vi "bluetooth com template.vi"   [LabVIEW 2021]
uses:
  <vilib>/Aledyne-TSXperts/Arduino Compatible Compiler for LabVIEW/Code Generator/Arduino APIs/Digital/PinDirection.ctl
  <vilib>/Aledyne-TSXperts/Arduino Compatible Compiler for LabVIEW/Code Generator/Arduino APIs/Serial/Serial Settings.ctl
  <vilib>/Aledyne-TSXperts/Arduino Compatible Compiler for LabVIEW/Arduino Compatible Compiler for LabVIEW.lvlib
types:
  T1 = typedef "Arduino Compatible Compiler for LabVIEW.lvlib/PinDirection.ctl" = enum16{" INPUT", "OUTPUT", " INPUT_PULLUP"}
  T2 = typedef "Arduino Compatible Compiler for LabVIEW.lvlib/Serial Settings.ctl" = u16
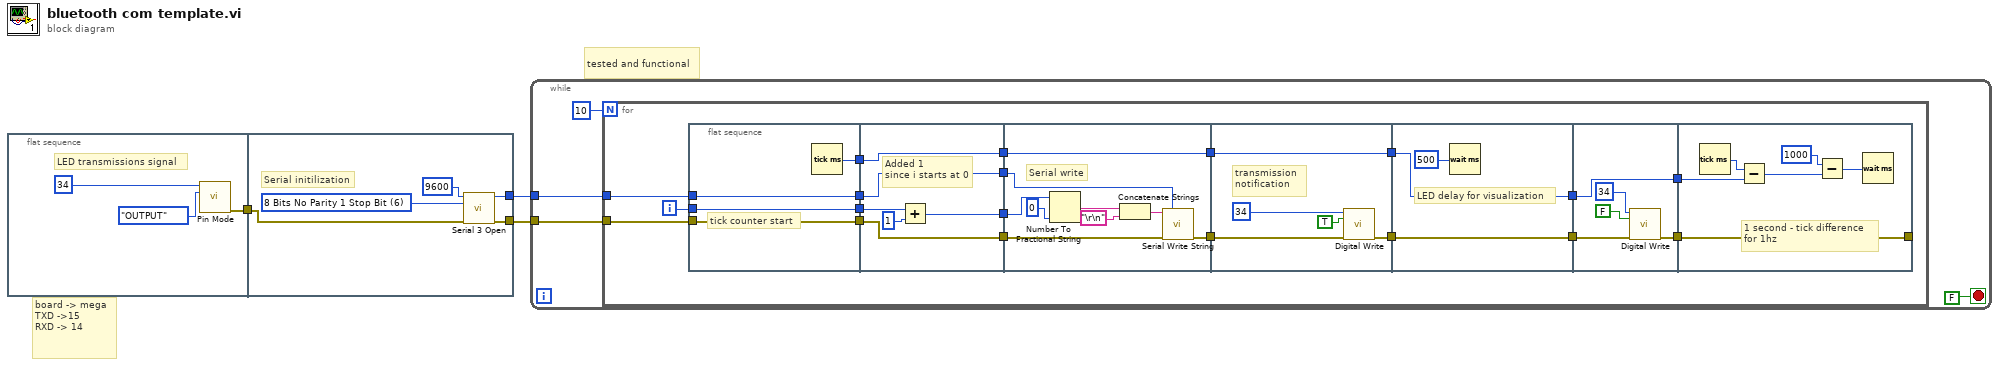
[diagram p0: block diagram]
diagram:
  # "tested and functional"
  # "board -> mega\nTXD ->15\nRXD -> 14"
  n1 = flat-sequence {
    tunnel: [w4] -> w3
    tunnel: [w11] -> w1
    tunnel: [w10] -> w2
    tunnel: w3 -> [w7]
    frame #0 {
      # "LED transmissions signal"
      n2 = call <vilib>:"Pin Mode.vi"("pin"=u8 34, "direction"=PinDirection."OUTPUT") -> ("error out"=w4:errorcluster)  [unwired: 13 in]
    }
    frame #1 {
      w8 = T2 6 items=["5 Bits No Parity 1 Stop Bit"=0, "6 Bits No Parity 1 Stop Bit"=2, "7 Bits No Parity 1 Stop Bit"=4, "8 Bits No Parity 1 Stop Bit"=6, "5 Bits No Parity 2 Stop Bits"=8, "6 Bits No Parity 2 Stop Bits"=10, "7 Bits No Parity 2 Stop Bits"=12, "8 Bits No Parity 2 Stop Bits"=14, "5 Bits Even Parity 1 Stop Bits"=32, "6 Bits Even Parity 1 Stop Bits"=34, "7 Bits Even Parity 1 Stop Bits"=36, "8 Bits Even Parity 1 Stop Bits"=38, "5 Bits Even Parity 2 Stop Bits"=40, "6 Bits Even Parity 2 Stop Bits"=42, "7 Bits Even Parity 2 Stop Bits"=44, "8 Bits Even Parity 2 Stop Bits"=46, "5 Bits Odd Parity 1 Stop Bits"=48, "6 Bits Odd Parity 1 Stop Bits"=50, "7 Bits Odd Parity 1 Stop Bits"=52, "8 Bits Odd Parity 1 Stop Bits"=54, "5 Bits Odd Parity 2 Stop Bits"=56, "6 Bits Odd Parity 2 Stop Bits"=58, "7 Bits Odd Parity 2 Stop Bits"=60, "8 Bits Odd Parity 2 Stop Bits"=62] ("Serial Settings")
      # "Serial initilization"
      n3 = call <vilib>:"Serial 3 Open.vi"("Speed"=u32 9600, "Serial Settings"=w8, "error in (no error)"=w7) -> ("Instance"=w10:u8, "error out"=w11:errorcluster)  [unwired: 11 in]
    }
  }
  n4 = while {
    tunnel: w2 -> [w15]
    tunnel: w1 -> [w14]
    stop <- FALSE stop-if-true
    n5 = for {
      N: 10 -> [_]
      tunnel: w15 -> [w34]
      tunnel: w14 -> [w33]
      i -> [w32]
      n6 = flat-sequence {
        tunnel: w33 -> [w36]
        tunnel: w34 -> [w37]
        tunnel: w32 -> [w38]
        tunnel: [w38] -> w25
        tunnel: [w37] -> w24
        tunnel: [w36] -> w23
        tunnel: [w35] -> w16
        tunnel: [w40] -> w28
        tunnel: [w44] -> w27
        tunnel: [w43] -> w26
        tunnel: w25 -> [w42]
        tunnel: w24 -> [w44]
        tunnel: w23 -> [w43]
        tunnel: [w39] -> w17
        tunnel: w16 -> [w39]
        tunnel: [w46] -> w31
        tunnel: w28 -> [w53]
        tunnel: w27 -> [w51]
        tunnel: w26 -> [w50]
        tunnel: [w45] -> w18
        tunnel: w17 -> [w45]
        tunnel: w31 -> [w56]
        tunnel: [w55] -> w29
        tunnel: [w54] -> w19
        tunnel: w18 -> [w54]
        tunnel: [w60] -> w30
        tunnel: w29 -> [w60]
        tunnel: [w59] -> w20
        tunnel: w19 -> [w59]
        tunnel: w30 -> [w64]
        tunnel: [w63] -> w22
        tunnel: [w62] -> w21
        tunnel: w20 -> [w62]
        tunnel: [w72] -> _
        tunnel: w22 -> [w72]
        tunnel: w21 -> [w67]
        frame #0 {
          # "tick counter start"
          n7 = Tick Count (ms)() -> (millisecond timer value=w35:u32)
        }
        frame #1 {
          # "Added 1\nsince i starts at 0"
          n8 = Add(x=w42, y=1) -> (x+y=w40:i32)
        }
        frame #2 {
          # "Serial write"
          n9 = Number To Fractional String(number=w53, precision (6)=i16 0) -> (F-format string=w48:string)  [unwired: 2 in]
          n10 = Concatenate Strings(w48, "\r\n") -> (w47:string)
          n11 = call <vilib>:"Serial Write String.vi"("String"=w47, "Instance"=w51, "error in (no error)"=w50) -> ("error out"=w46:errorcluster)  [unwired: 12 in]
        }
        frame #3 {
          # "transmission \nnotification"
          n12 = call <vilib>:"Digital Write.vi"("pin"=u8 34, "state"=TRUE, "error in (no error)"=w56) -> ("error out"=w55:errorcluster)  [unwired: 12 in]
        }
        frame #4 {
          # "LED delay for visualization"
          n13 = Wait (ms)(milliseconds to wait=u32 500) -> ()  [unwired: 1 out]
        }
        frame #5 {
          n14 = call <vilib>:"Digital Write.vi"("pin"=u8 34, "state"=FALSE, "error in (no error)"=w64) -> ("error out"=w63:errorcluster)  [unwired: 12 in]
        }
        frame #6 {
          # "1 second - tick difference\nfor 1hz"
          n15 = Tick Count (ms)() -> (millisecond timer value=w68:u32)
          n16 = Subtract(x=w68, y=w67) -> (x-y=w71:u32)
          n17 = Subtract(x=u32 1000, y=w71) -> (x-y=w69:u32)
          n18 = Wait (ms)(milliseconds to wait=w69) -> ()  [unwired: 1 out]
        }
      }
    }
  }
